vi "Build Frame Instructions.vi"(7 "Virtual Memory Unit in":refnum<class "Virtual Memory Unit.lvclass">, 8 "error in (no error)":errorcluster, 9 "Message Pointers":T1 {"HP Async Address" format="%04x"; "SubRoutine Address" format="%04x"}, 10 "Starting Address":u16 format="%04x", 11 "Message in":refnum<class "Message.lvclass">) -> (0 "error out":errorcluster, 1 "Msg Already Configured":bool, 2 "Next Available Address":u16 format="%04x", 3 "Message out":refnum<class "Message.lvclass">, 5 "Virtual Memory Unit out":refnum<class "Virtual Memory Unit.lvclass">)   [LabVIEW 2020, in "BCI-1553 API.lvlib" / "Message.lvclass"]
doc: "<DO NOT CALL>\n\nBuilds the instructions for executing a message. If a message has already been configured with an address pointer, reuse the existing pointer. This makes sure all copies of this message + ID pair will refer to the same block of memory."
uses:
  Message.lvclass
  Dependencies/Virtual Memory Unit/Virtual Memory Unit.lvclass
  TypeDefs/Message Pointers.ctl
  TypeDefs/BC Op Codes - Verbose.ctl
  TypeDefs/BC Condition Codes.ctl
  Message.lvclass/Message.ctl
  BCI-1553 API.lvlib
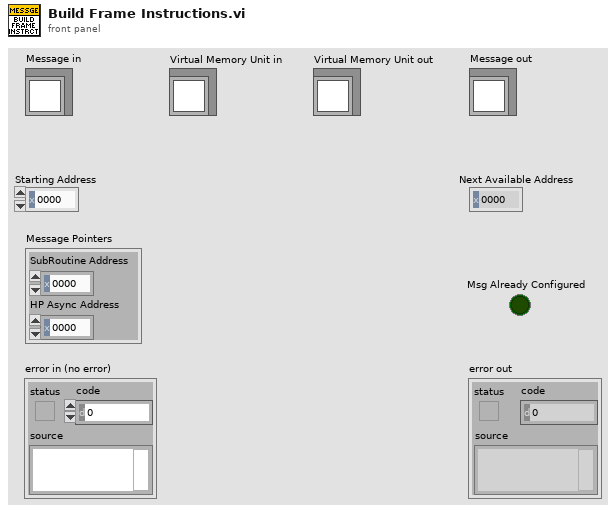
[diagram p1: front panel]
types:
  T1 = typedef "BCI-1553 API.lvlib/Message Pointers.ctl" = cluster{"SubRoutine Address":u16, "HP Async Address":u16}
  T2 = typedef "BCI-1553 API.lvlib/BC Condition Codes.ctl" = enum16{"GP0 == 1 || LT", "GP1 == 1 || NE", "GP2 == 1", "GP3 == 1", "GP4 == 1", "GP5 == 1", "GP6 == 1", "GP7 == 1", "NORESP", "FMTERR", "GOODBLOCK", "MSKSTATSET", "BADMSG", "1RETRY", "2RETRY", "ALWAYS"}
  T3 = typedef "BCI-1553 API.lvlib/BC Op Codes - Verbose.ctl" = enum16{"EXECUTE MSG", "EXECUTE MSG GO", "JUMP", "CALL SUBROUTINE", "RETURN", "INTERRUPT REQUEST", "HALT", "DELAY", "WAIT FRAME TIMER = 0", "COMPARE FRAME TIMER", "COMPARE MSG TIMER", "LOAD TIME TAG CTR", "LOAD TIME TAG CTR HI", "LOAD FRAME TIMER", "START FRAME TIMER", "PUSH TIME TAG COUNT", "PUSH TIME TAG COUNT HI", "PUSH TIME TAG COUNT BOTH", "PUSH BLOCK STATUS WORD", "PUSH CURRENT VALUE", "PUSH INDIRECT", "WAIT EXT TRIGGER", "EXECUTE AND FLIP", "EXECUTE, FLIP, GO", "WRITE VALUE TO WMI", "WRITE VALUE TO MEM", "DECREMENT RAM, SKIP", "FLAG"}
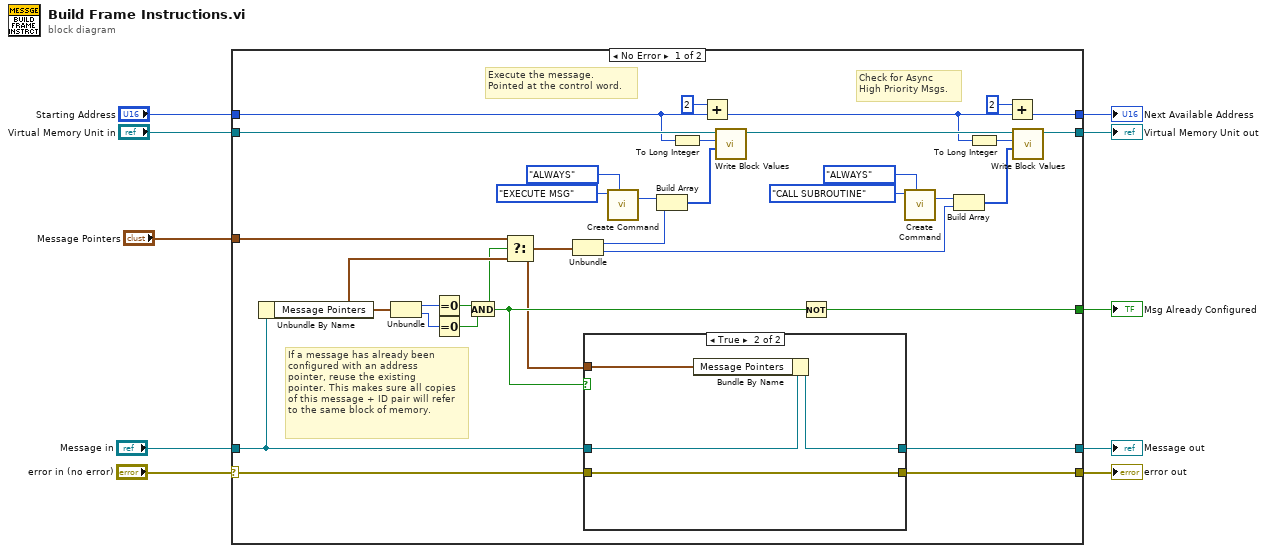
[diagram p0: block diagram]
diagram:
  n1 = case shown="No Error" "error in (no error)" {
    selector: "error in (no error)" -> [w15 w53]
    tunnel: [w12 w53] -> w9
    tunnel: [w14 w52] -> w7
    tunnel: "Message in" -> [w13 w52]
    tunnel: "Starting Address" -> [w41 w51]
    tunnel: "Virtual Memory Unit in" -> [w42 w50]
    tunnel: [w25 w51] -> w4
    tunnel: [w27 w50] -> w3
    tunnel: "Message Pointers" -> [w19 _]
    tunnel: [w17 _] -> w1
    frame No Error {
      # "If a message has already been\nconfigured with an address\npointer, reuse the existing\npointer. This makes sure all copies\nof this message + ID pair will refer\nto the same block of memory."
      # "Check for Async\nHigh Priority Msgs."
      # "Execute the message.\nPointed at the control word."
      n2 = Unbundle By Name(w13) -> ("Message Pointers"=w18:T1)
      n3 = Unbundle(w18) -> ("SubRoutine Address"=w23:u16, "HP Async Address"=w22:u16)
      n4 = Equal To 0?(x=w23) -> (x = 0?=w20:bool)
      n5 = Equal To 0?(x=w22) -> (x = 0?=w21:bool)
      n6 = And(x=w20, y=w21) -> (x .and. y?=w16:bool)
      n7 = Select(t=w19, s=w16, f=w18) -> (s? t:f=w11:T1)
      n8 = Unbundle(w11) -> ("SubRoutine Address"=w35:u16, "HP Async Address"=w24:u16)
      n9 = case shown="True" w16 {
        tunnel: w15 -> [w44 w49]
        tunnel: [w45 w47] -> w14
        tunnel: w13 -> [w45 w48]
        tunnel: [w44 w49] -> w12
        tunnel: w11 -> [_ w46]
        frame False {
        }
        frame True {
          n10 = Bundle By Name(cluster=w48, "Message Pointers"=w46) -> (w47:refnum<class "Message.lvclass">)
        }
      }
      n11 = call "Create Command.vi"("Condition"=BC_Condition_Codes."ALWAYS", "Op Code"=BC_Op_Codes_-_Verbose."EXECUTE MSG") -> ("Instruction"=w37:u16)  [unwired: 8 in, 1 out]
      n12 = Build Array(w37, w35) -> (w36:u16[])
      n13 = To Long Integer(number=w41) -> (32bit integer=w40:i32)
      n14 = Add(x=u16 2, y=w41) -> (x+y=w26:u16)
      n15 = call "Write Block Values.vi"("Write Block"=w36, "Start Index"=w40, "Virtual Memory Unit in"=w42) -> ("Virtual Memory Unit out"=w28:refnum<class "Virtual Memory Unit.lvclass">)  [unwired: 7 in, 1 out]
      n16 = Not(x=w16) -> (.not. x?=w17:bool)
      n17 = call "Create Command.vi"("Condition"=BC_Condition_Codes."ALWAYS", "Op Code"=BC_Op_Codes_-_Verbose."CALL SUBROUTINE") -> ("Instruction"=w33:u16)  [unwired: 8 in, 1 out]
      n18 = Build Array(w33, w24) -> (w34:u16[])
      n19 = To Long Integer(number=w26) -> (32bit integer=w30:i32)
      n20 = Add(x=u16 2, y=w26) -> (x+y=w25:u16)
      n21 = call "Write Block Values.vi"("Write Block"=w34, "Start Index"=w30, "Virtual Memory Unit in"=w28) -> ("Virtual Memory Unit out"=w27:refnum<class "Virtual Memory Unit.lvclass">)  [unwired: 7 in, 1 out]
    }
    frame Error {
    }
  }
  "error out" <- w9
  "Message out" <- w7
  "Virtual Memory Unit out" <- w3
  "Next Available Address" <- w4
  "Msg Already Configured" <- w1
